vi "Run_on_Start.vi"(11 "val in":sgl) -> (3 "Val out":sgl)   [LabVIEW 2014]
uses:
  Start.vi
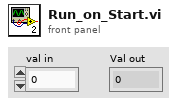
[diagram p1: front panel]
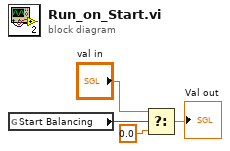
[diagram p0: block diagram]
diagram:
  n1 = global read "Start.vi" "Start Balancing"() -> (w1:bool)
  n2 = Select(t="val in", s=w1, f=sgl 0.0) -> (s? t:f=→"Val out":sgl)
